vi "FTW-TransferClient-S3-SetHeaders.vi"(0 "Headers":refnum<k24>, 5 "Headers Collection":T1[](array[typedef])=[{"Key"="Content-Type", "Value"="application/octet-stream"}], 11 "error in":errorcluster) -> (15 "error out":errorcluster)   [LabVIEW 2014, in "FTW-TransferClient-S3.lvclass"]
uses:
  FTW-TransferClient-S3.lvclass
  sandbox/deprecated/FTW-Collection-KeyValuePair.ctl
  C:/Users/Jack/repo/ftw-master/ftw/src/windows/transfer/S3/AWSSDK.dll
  AWSSDK.dll
panel:
  # "Inputs"
  # "Outputs"
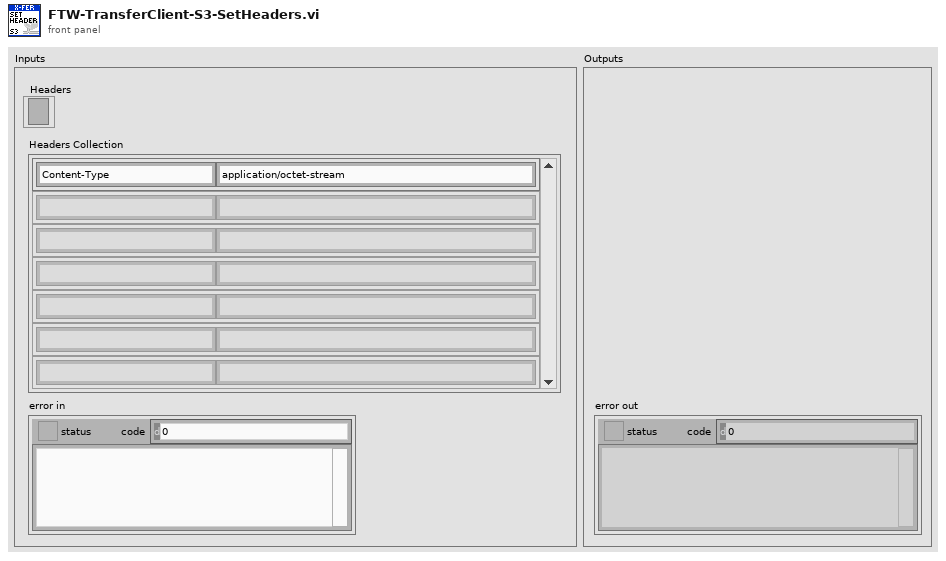
[diagram p1: front panel]
types:
  T1 = typedef "FTW-Collection-KeyValuePair.ctl" = cluster{"Key":string, "Value":string}
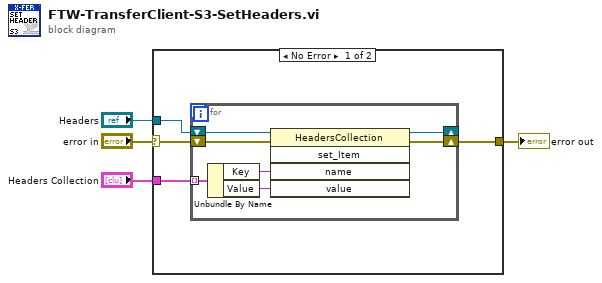
[diagram p0: block diagram]
diagram:
  n1 = case shown="No Error" "error in" {
    selector: "error in" -> [w6 w16]
    tunnel: [w7 w16] -> w4
    tunnel: "Headers Collection" -> [w8 _]
    tunnel: "Headers" -> [w5 _]
    frame No Error {
      n2 = for {
        shift-right: [w12] -> _
        shift-left: w5 -> [w15]
        shift-right: [w13] -> w7
        shift-left: w6 -> [w14]
        tunnel: w8 -> [w11] mode=indexing
        n3 = Unbundle By Name(w11) -> ("Key"=w10:string, "Value"=w9:string)
        n4 = invoke class="HeadersCollection" method="set_Item"(reference=w15, error in=w14, "name"=w10, "value"=w9) -> (reference out=w12:refnum<k24>, error out=w13:errorcluster)  [unwired: 1 in, 3 out]
      }
    }
    frame Error {
    }
  }
  "error out" <- w4
